vi "init.vi"(8 "error in (no error)":errorcluster, 10 "Variant":variant, 11 "PSP-603 in":refnum<class "PSP-603.lvclass">) -> (0 "error out":errorcluster, 3 "PSP-603 out":refnum<class "PSP-603.lvclass">)   [LabVIEW 2025, in "Power Supply.lvlib" / "PSP-603.lvclass"]
uses:
  PSP-603.lvclass
  PSP-603.lvclass/PSP-603.ctl
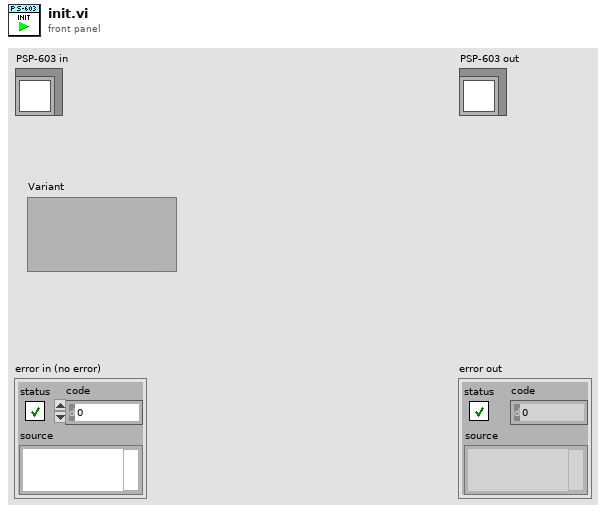
[diagram p1: front panel]
types:
  T1 = cluster{"Baud_Rate":u16, "Data_Bits":u16, "Parity":u16, "Stop_Bits":u16, "Flow_Control":u16, "Termination_Char":u8, "Receive Termination Char?":bool, "Send Termination Char?":bool}
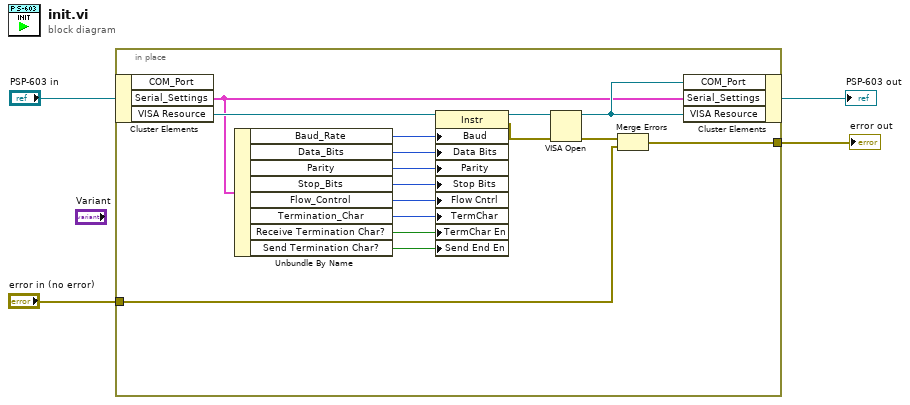
[diagram p0: block diagram]
diagram:
  n1 = in-place {
    in-place-border: [w5] -> w2
    in-place-border: "error in (no error)" -> [w6]
    n2 = in-place-cluster #1("PSP-603 in") -> ("Serial_Settings"=w8:T1, "VISA Resource"=w20:refnum<visa-resource-name>)  [unwired: 1 out]
    n3 = Unbundle By Name(w8) -> ("Baud_Rate"=w19:u16, "Data_Bits"=w18:u16, "Parity"=w17:u16, "Stop_Bits"=w16:u16, "Flow_Control"=w15:u16, "Termination_Char"=w14:u8, "Receive Termination Char?"=w13:bool, "Send Termination Char?"=w12:bool)
    n4 = property class="Instr"(reference=w20, "Baud"=w19, "Data Bits"=w18, "Parity"=w17, "Stop Bits"=w16, "Flow Cntrl"=w15, "TermChar"=w14, "TermChar En"=w13, "Send End En"=w12) -> (reference out=w11:refnum<visa-resource-name>, error out=w10:errorcluster)  [unwired: 1 in]
    n5 = VISA Open(error in (no error)=w10, VISA resource name=w11) -> (VISA resource name=w9:refnum<visa-resource-name>, error out=w7:errorcluster)  [unwired: 3 in]
    n6 = Merge Errors(w7, w6) -> (w5:errorcluster)
    n7 = in-place-cluster #1("COM_Port"=w9, "Serial_Settings"=w8, "VISA Resource"=w9) -> (→"PSP-603 out":refnum<class "PSP-603.lvclass">)
  }
  "error out" <- w2
